vi "Read Unique ID.vi"(11 "IObserver In":refnum<class "IObserver.lvclass">) -> (2 "Unique ID":string)   [LabVIEW 2020, in "IObserver.lvlib" / "IObserver.lvclass"]
doc: "读取 Actor 队列 DVR 引用唯一 ID"
uses:
  IObserver.lvclass
  IObserver.lvclass/IObserver.ctl
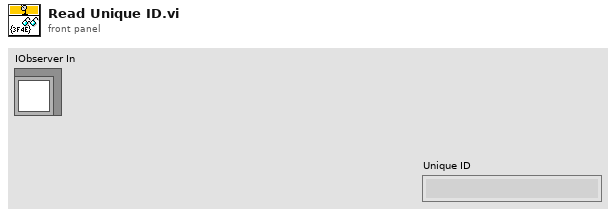
[diagram p1: front panel]
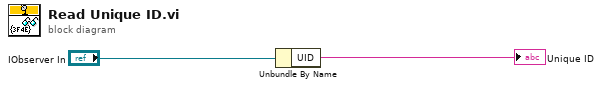
[diagram p0: block diagram]
diagram:
  n1 = Unbundle By Name("IObserver In") -> ("UID"=→"Unique ID":string)
